vi "ConvertArrayToMessages.vi"(8 "error in (no error)":errorcluster, 11 "Array":bool[][](array[boolean])=array64x128[8192 elements]) -> (0 "error out":errorcluster, 3 "Messages":string[](array[string]))   [LabVIEW 2020, in "CTI-Peripheral.lvlib" / "64x128 I2C OLED SSD1315.lvclass"]
uses:
  64x128 I2C OLED SSD1315.lvclass
  64x128 I2C OLED SSD1315.lvclass/64x128 I2C OLED SSD1315.ctl
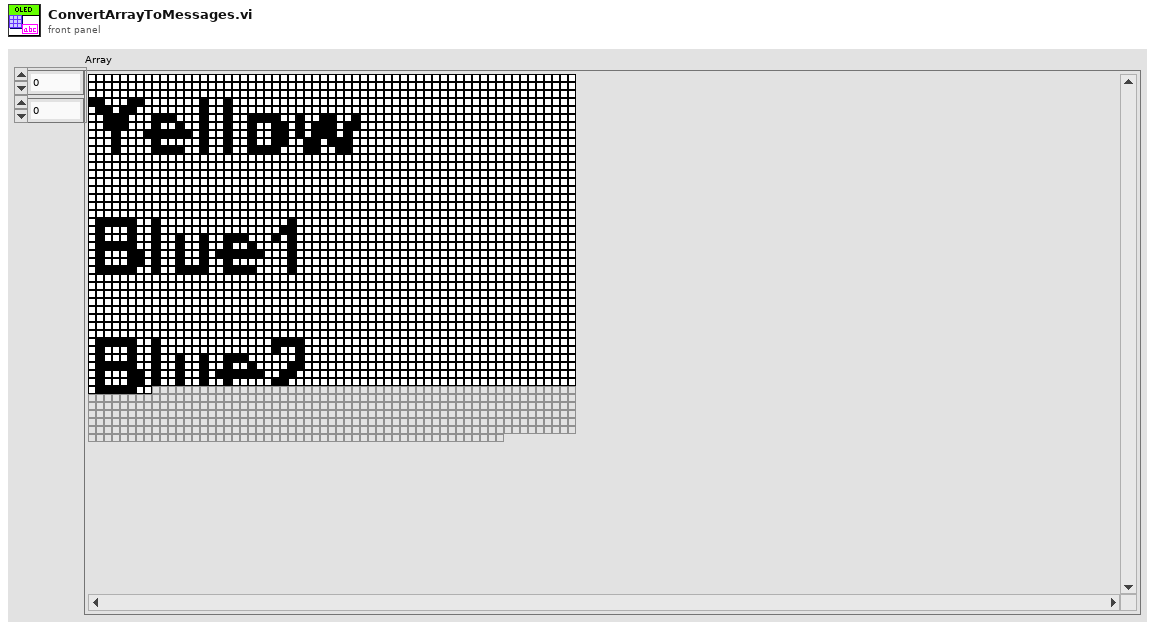
[diagram p1: front panel]
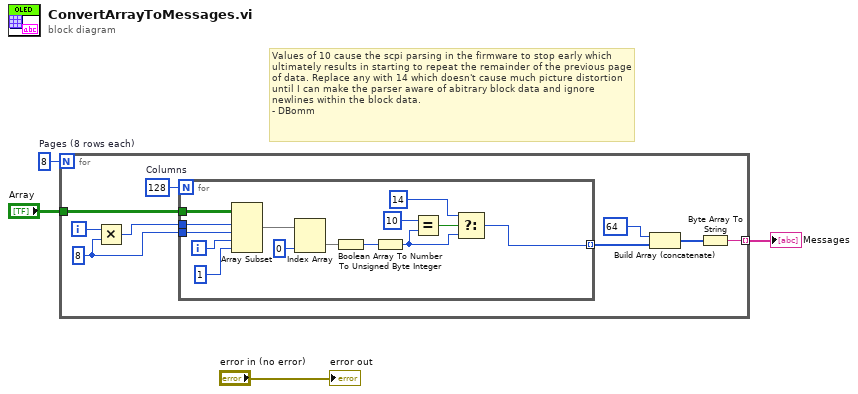
[diagram p0: block diagram]
diagram:
  w3 = 8  # Pages (8 rows each)
  # "Values of 10 cause the scpi parsing in the firmware to stop early which ultimately results in starting to repeat the remainder of the previous page of data. Replace any with 14 which doesn't cause much picture distortion until I can make the parser aware of abitrary block data and ignore newlines within the block data.\n- DBomm"
  n1 = for {
    N: w3 -> [_]
    tunnel: "Array" -> [w13]
    tunnel: [w5] -> w1 mode=indexing
    i -> [w12]
    w9 = 128  # Columns
    w10 = 8 ("y")
    n2 = Multiply(x=w12, y=w10) -> (x*y=w11:i32)
    n3 = for {
      N: w9 -> [_]
      tunnel: w13 -> [w27]
      tunnel: w11 -> [w26]
      tunnel: w10 -> [w25]
      tunnel: [w14] -> w8 mode=indexing
      i -> [w24]
      n4 = Array Subset(array=w27, index (row)=w26, length (row)=w25, index (col)=w24, length (col)=1 ("length")) -> (w22:bool[][])
      n5 = Index Array(array=w22, index (col)=0 ("disabled index (col)")) -> (element=w20:bool[])  [unwired: 1 in]
      n6 = Boolean Array To Number(Boolean array=w20) -> (number=w19:u32)
      n7 = To Unsigned Byte Integer(number=w19) -> (unsigned 8bit integer=w15:u8)
      n8 = Equal?(x=u8 10, y=w15) -> (x = y?=w17:bool)
      n9 = Select(t=u8 14 ("x"), s=w17, f=w15) -> (s? t:f=w14:u8)
    }
    n10 = Build Array (concatenate)(u8 64 ("element"), w8) -> (w6:u8[])
    n11 = Byte Array To String(unsigned byte array=w6) -> (string=w5:string)
  }
  "Messages" <- w1
  "error out" <- "error in (no error)"
